vi "LoadController.vi"(8 "error in (no error)":errorcluster, 10 "Actor In":refnum<class "Actor.lvclass">, 11 "DemoMicrosope in":refnum<class "DemoMicrosope.lvclass">) -> (0 "error out":errorcluster, 3 "DemoMicrosope out":refnum<class "DemoMicrosope.lvclass">)   [LabVIEW 2020, in "DemoMicrosope.lvlib" / "DemoMicrosope.lvclass"]
uses:
  DemoMicrosope.lvclass
  <vilib>/ActorFramework/Actor/Actor.lvclass
  ViewController/Microscope Controller/MicroscopeController.lvclass
  C:/Program Files/National Instruments/LabVIEW 2020/vi.lib/ActorFramework/Actor/Actor.lvclass
  Hardware Abstraction Layer/Microscope/Microscope/Microscope.lvclass
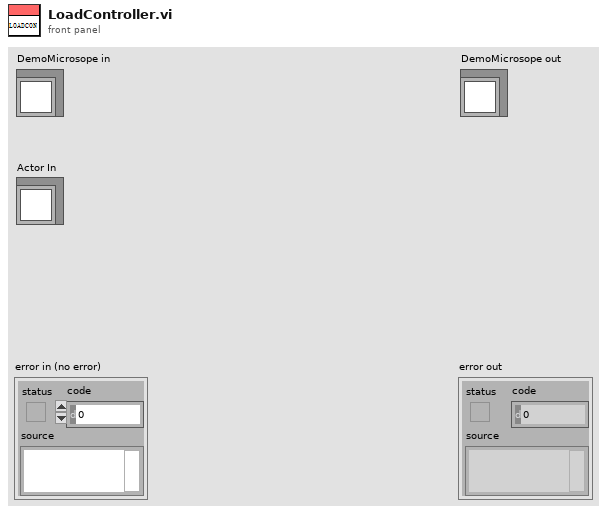
[diagram p1: front panel]
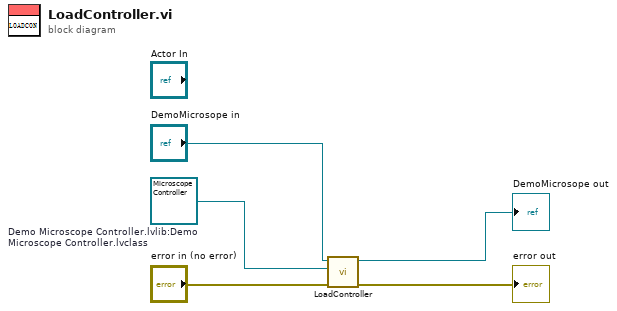
[diagram p0: block diagram]
diagram:
  w3 = refnum<class "MicroscopeController.lvclass"> refnum  # Demo Microscope Controller.lvlib:Demo Microscope Controller.lvclass
  n1 = call-parent "LoadController.vi"("error in (no error)"="error in (no error)", "Actor In"=w3, "Microscope in"="DemoMicrosope in") -> ("error out"=→"error out":errorcluster, "Microscope out"=→"DemoMicrosope out":refnum<class "DemoMicrosope.lvclass">)  [unwired: 7 in]
